vi "Photon Counter with LCD Reader.vi"(8 "error in (no error)":errorcluster, 10 "Photon Counter in":refnum<class "Photon Counter.lvclass">, 11 "Photon Counter with LCD Reader in":refnum<class "Photon Counter with LCD Reader.lvclass">) -> (0 "error out":errorcluster, 3 "Photon Counter with LCD Reader out":refnum<class "Photon Counter with LCD Reader.lvclass">)   [LabVIEW 2023, in "Photon Counter with LCD Reader.lvclass"]
uses:
  Photon Counter with LCD Reader.lvclass
  C:/LabVIEW-programs/Readers/Reader/Reader.lvclass
  Instruments/Photon Counter/Photon Counter.lvclass
  C:/LabVIEW-programs/Instruments/Utility Classes/Readable/Readable.lvclass
  Photon Counter with LCD Reader.lvclass/Photon Counter with LCD Reader.ctl
  Reader/Reader.lvclass
  Instruments/LCD/LCD Retarder.lvclass
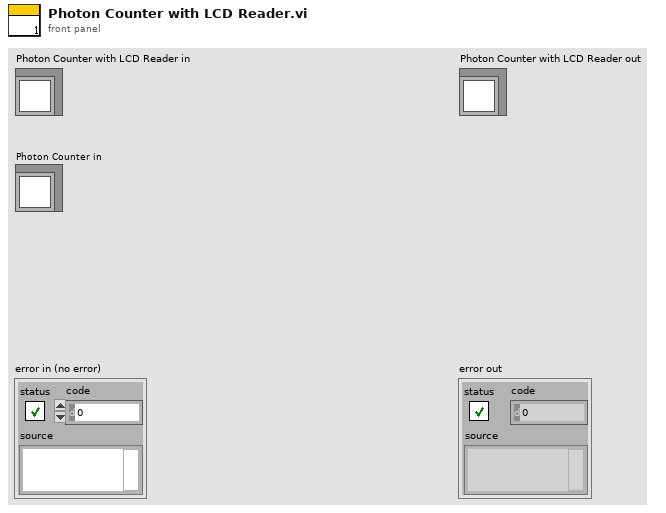
[diagram p1: front panel]
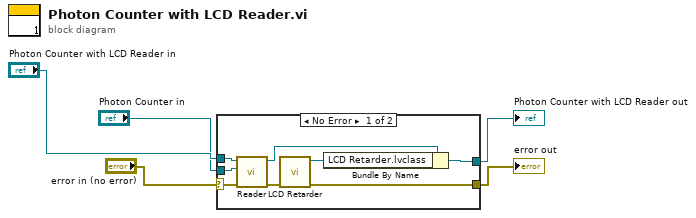
[diagram p0: block diagram]
diagram:
  n1 = case shown="No Error" "error in (no error)" {
    selector: "error in (no error)" -> [w12 w15]
    tunnel: [w9 w15] -> w4
    tunnel: [w8 w14] -> w2
    tunnel: "Photon Counter with LCD Reader in" -> [w13 w14]
    tunnel: "Photon Counter in" -> [w11 _]
    frame No Error {
      n2 = call "Reader.vi"("error in (no error)"=w12, "Readable"=w11, "Reader in"=w13) -> ("error out"=w10:errorcluster, "Reader out"=w7:refnum<class "Photon Counter with LCD Reader.lvclass">)  [unwired: 7 out]
      n3 = call "LCD Retarder.vi"("error in"=w10) -> ("errorOUT"=w9:errorcluster, "LCD out"=w6:refnum<class "LCD Retarder.lvclass">)  [unwired: 9 in]
      n4 = Bundle By Name(cluster=w7, "LCD Retarder.lvclass"=w6) -> (w8:refnum<class "Photon Counter with LCD Reader.lvclass">)
    }
    frame Error {
    }
  }
  "error out" <- w4
  "Photon Counter with LCD Reader out" <- w2
